vi "time_step_attempt.vi"() -> ()   [LabVIEW 2017]
panel:
  in  "Time to hold at start value":dbl
  out "Current value":i32
  in  "Number of cycles":i32
  out "Number of steps":i32
  out "Number of cycles":i32
  in  "End value":i32
  in  "Start value":i32
  in  "Step value":i32
  in  "Seconds between steps":dbl
  in  "stop":bool
  out "current ref time":timestamp
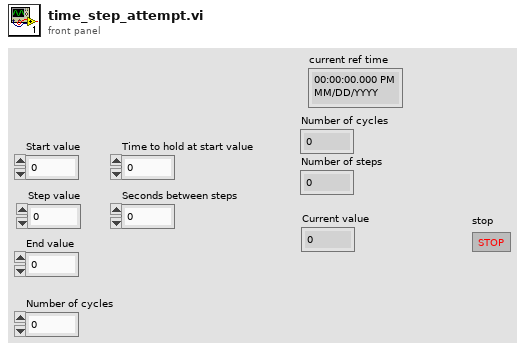
[diagram p1: front panel]
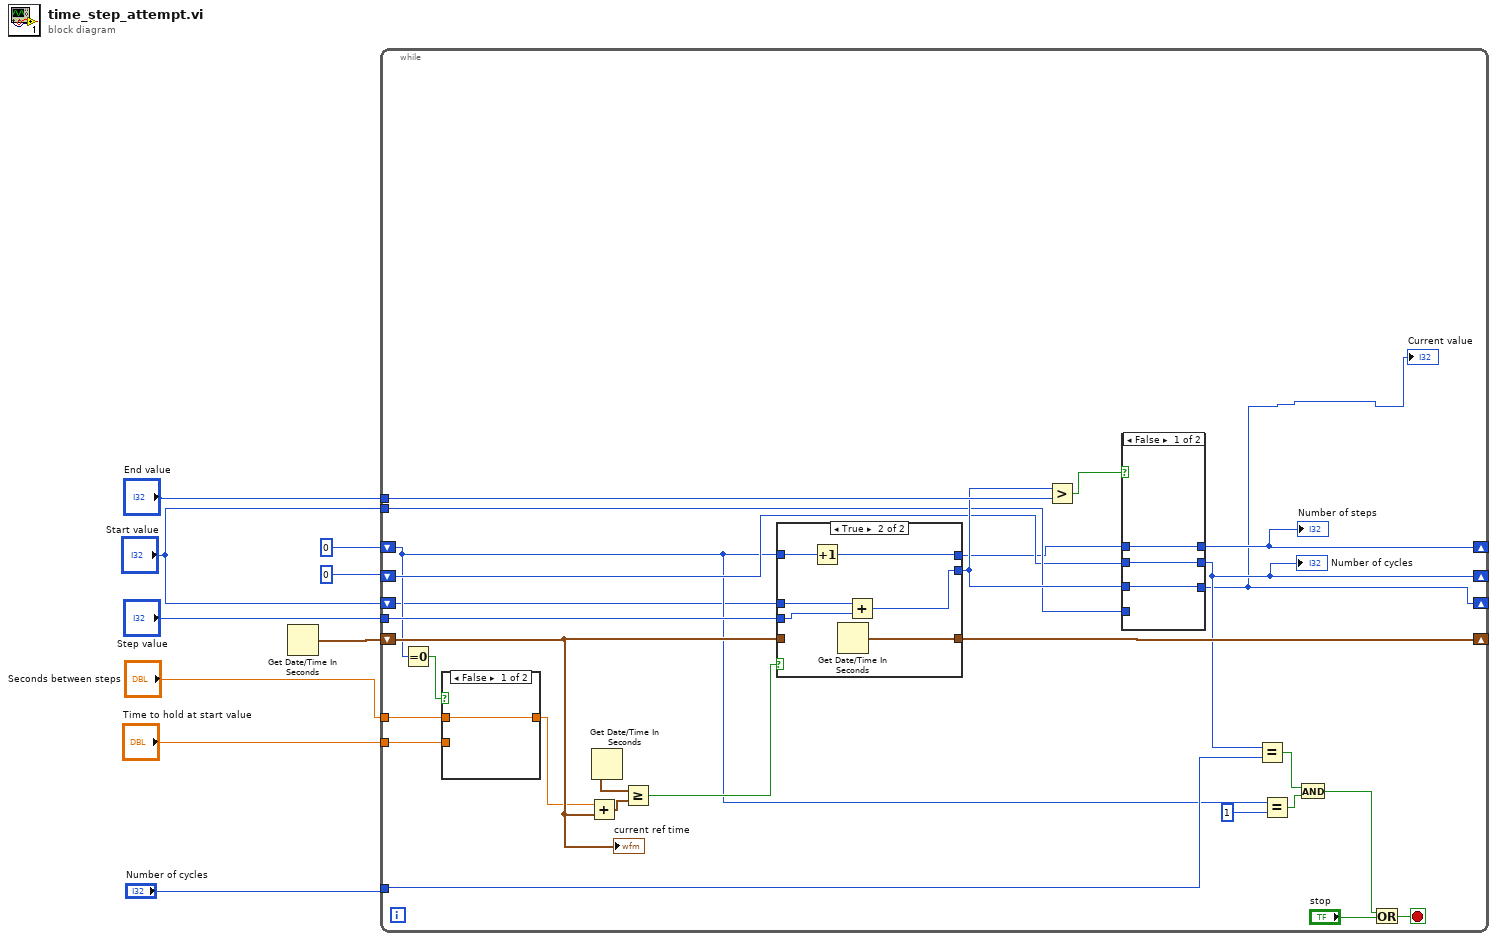
[diagram p0: block diagram]
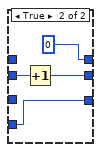
[diagram p3: hidden frame]
diagram:
  n1 = Get Date/Time In Seconds() -> (seconds since 1Jan1904=w8:timestamp)
  n2 = while {
    shift-right: [w10] -> _
    shift-left: "Start value" -> [w13]
    tunnel: "Step value" -> [w34]
    shift-right: [w33] -> _
    shift-left: w8 -> [w32]
    tunnel: "Seconds between steps" -> [w18]
    shift-right: [w22] -> _
    shift-left: 0 -> [w16]
    tunnel: "End value" -> [w31]
    tunnel: "Start value" -> [w28]
    shift-right: [w26] -> _
    shift-left: 0 -> [w27]
    tunnel: "Number of cycles" -> [w25]
    tunnel: "Time to hold at start value" -> [w19]
    stop <- w11 stop-if-true
    n3 = Equal To 0?(x=w16) -> (x = 0?=w21:bool)
    n4 = case shown="False" w21 {
      tunnel: [w38 w39] -> w20
      tunnel: w19 -> [_ w39]
      tunnel: w18 -> [w38 _]
      frame False {
      }
      frame True {
      }
    }
    n5 = Add(x=w20, y=w32) -> (x+y=w37:timestamp)
    n6 = Get Date/Time In Seconds() -> (seconds since 1Jan1904=w36:timestamp)
    n7 = Greater Or Equal?(x=w36, y=w37) -> (x >= y?=w35:bool)
    n8 = case shown="True" w35 {
      tunnel: w13 -> [w49 w55]
      tunnel: [w49 w53] -> w29
      tunnel: w34 -> [_ w54]
      tunnel: [w47 w52] -> w33
      tunnel: [w48 w51] -> w23
      tunnel: w16 -> [w48 w50]
      tunnel: w32 -> [w47 _]
      frame False {
      }
      frame True {
        n9 = Increment(x=w50) -> (x+1=w51:i32)
        n10 = Get Date/Time In Seconds() -> (seconds since 1Jan1904=w52:timestamp)
        n11 = Add(x=w55, y=w54) -> (x+y=w53:i32)
      }
    }
    n12 = Greater?(x=w29, y=w31) -> (0:w30:bool)
    n13 = case shown="False" w30 {
      tunnel: w29 -> [w42 _]
      tunnel: [w42 w46] -> w10
      tunnel: w28 -> [_ w46]
      tunnel: [w41 w45] -> w26
      tunnel: w27 -> [w41 w44]
      tunnel: w23 -> [w40 _]
      tunnel: [w40 0] -> w22
      frame False {
      }
      frame True {
        n14 = Increment(x=w44) -> (x+1=w45:i32)
      }
    }
    "Number of cycles" <- w26
    "Number of steps" <- w22
    "Current value" <- w10
    n15 = Equal?(x=w26, y=w25) -> (x = y?=w17:bool)
    n16 = Equal?(x=w16, y=1) -> (x = y?=w14:bool)
    n17 = And(x=w17, y=w14) -> (x .and. y?=w12:bool)
    n18 = Or(x=w12, y="stop") -> (x .or. y?=w11:bool)
    "current ref time" <- w32
  }
